vi "Thorlabs MLJ - Z Stage Module.vi"(7 "Set/Get":T3=enum."Get", 8 "Error In":errorcluster, 10 "Action":T4=enum."Stop", 11 "Cluster In":T1={"Position"=0.0, "Is.Enabled?"=FALSE, "Is.Connected?"=FALSE, "Device SN"="45876539", "AccelerationMaximum"=0.0, "VelocityMaximum"=0.0, "Acceleration"=0.0, "Velocity"=0.0, "waitTimeout (ms)"=0, "Model"=enum."None", "Is.Homed?"=FALSE}) -> (0 "Error Out":errorcluster, 3 "Cluster Out":T1={"Position"=0.0, "Is.Enabled?"=FALSE, "Is.Connected?"=FALSE, "Device SN"="45876539", "AccelerationMaximum"=0.0, "VelocityMaximum"=0.0, "Acceleration"=0.0, "Velocity"=0.0, "waitTimeout (ms)"=0, "Model"=enum."None", "Is.Homed?"=FALSE})   [LabVIEW 2018]
uses:
  Controls/Motion Translation Module Control.ctl
  Controls/Translation Stage Cluster.ctl
  General/Controls/Translation Stage Types.ctl
  General/Controls/Set Get Controls.ctl
  C:/Project/SerialSectOCT/SerialSectOCT/Software/Thorlabs.MotionControl.Controls.dll
  Thorlabs.MotionControl.Controls.dll
panel:
  in  "MLJ Reference":refnum<k24>(container)
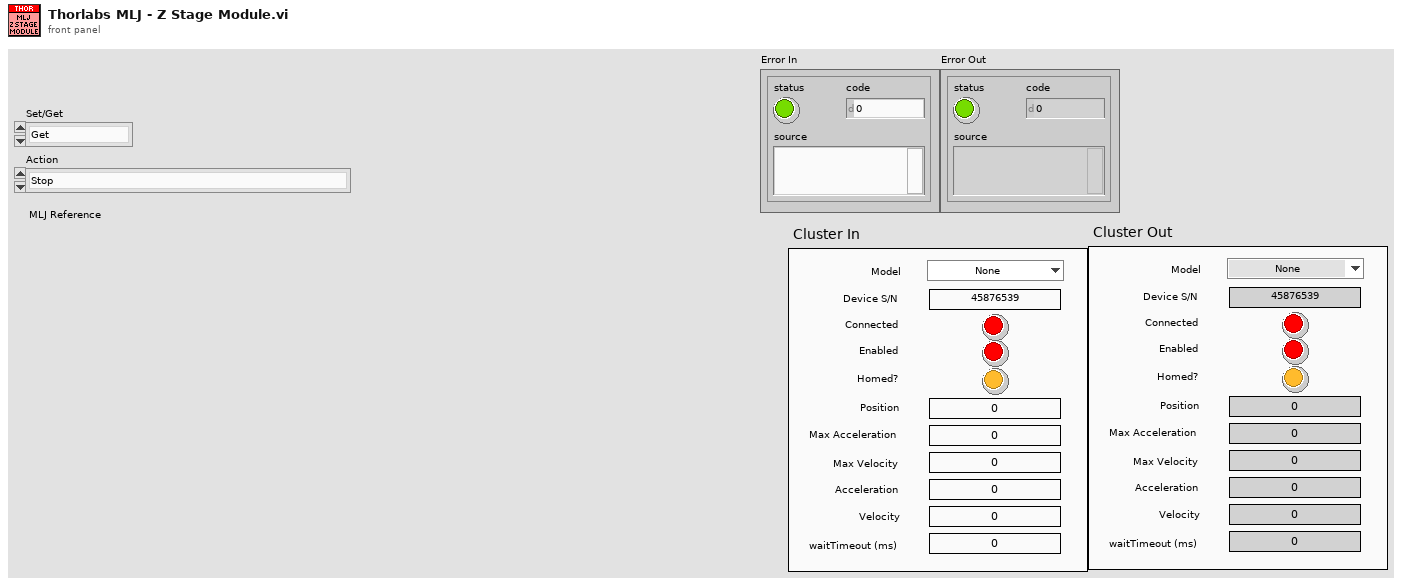
[diagram p1: front panel]
types:
  T1 = typedef "Translation Stage Cluster.ctl" = cluster{"Position":dbl, "Is.Enabled?":bool, "Is.Connected?":bool, "Device SN":string, "AccelerationMaximum":dbl, "VelocityMaximum":dbl, "Acceleration":dbl, "Velocity":dbl, "waitTimeout (ms)":i32, "Model":T2, "Is.Homed?":bool}
  T2 = typedef "Translation Stage Types.ctl" = enum16{"None", "Thorlabs LTS", "Thorlabs MLJ"}
  T3 = typedef "Set Get Controls.ctl" = enum16{"Set", "Get"}
  T4 = typedef "Motion Translation Module Control.ctl" = enum16{"Init", "Home", "Status", "Velocity/Accel", "Position", "Jog", "Stop", "Uninit", "Enable", "Disable"}
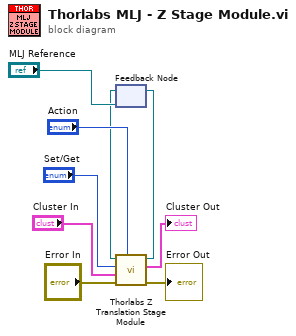
[diagram p0: block diagram]
diagram:
  n1 = feedback #1("MLJ Reference") -> (w1:refnum<k24>)
  n2 = call "Thorlabs Z Translation Stage Module.vi"("Action"="Action", "error in (no error)"="Error In", "Cluster In"="Cluster In", "Set/Get"="Set/Get", ".NET Refnum in"=w1) -> ("error out"=→"Error Out":errorcluster, "Cluster out"=→"Cluster Out":T1, ".NET Refnum out"=w3:refnum<k24>)  [unwired: 4 in]
  n3 = feedback-in #1(w3) -> ()
